vi "Initilaize Views.vi"(8 "error in (no error)":errorcluster, 11 "Example Source in":refnum<class "Example Controller Actor.lvclass">) -> (0 "error out":errorcluster, 3 "Example Source out":refnum<class "Example Controller Actor.lvclass">)   [LabVIEW 2016, in "Example Controller Actor.lvlib" / "Example Controller Actor.lvclass"]
uses:
  Example Controller Actor.lvclass
  C:/Projects/Shared Libraries/Event Actors/Controller Actor/Controller Actor.lvclass
  Example View Actor/Example View Actor/Example View Actor.lvclass
  C:/Projects/Shared Libraries/Event Actors/View Actor/View Actor.lvclass
  View Actor/View Actor.lvclass/View Actor.ctl
  View Actor/properties/Write Name.vi
  Controller Actor/Controller Actor.lvclass
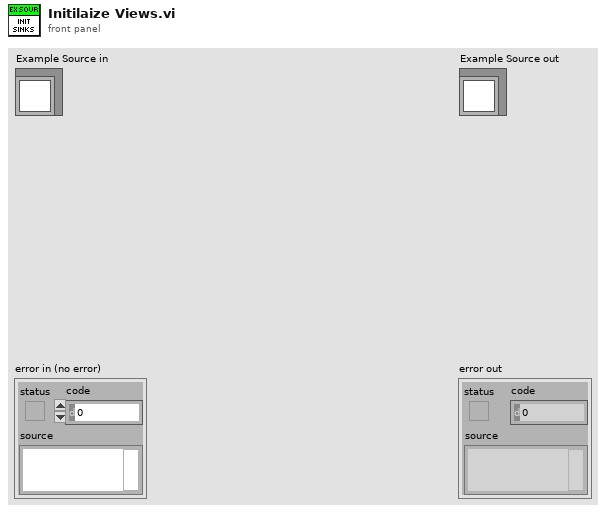
[diagram p1: front panel]
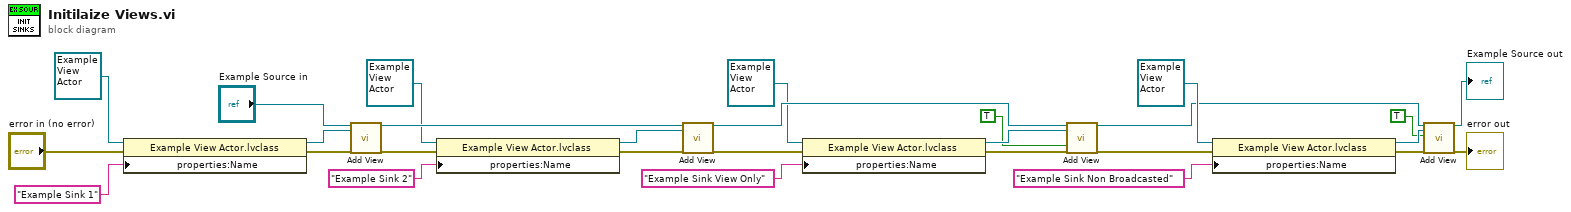
[diagram p0: block diagram]
diagram:
  n1 = property class="Example View Actor.lvclass"(reference=refnum<class "Example View Actor.lvclass"> refnum ("Alternative Example Sink.lvlib:Alternative Example Sink.lvclass"), error in="error in (no error)", "properties:Name"="Example Sink 1" ("Debug Alias")) -> (reference out=w27:refnum<class "Example View Actor.lvclass">, error out=w24:errorcluster)
  n2 = call "Add View.vi"("Controller Actor in"="Example Source in", "View Actor"=w27, "error in (no error)"=w24) -> ("Controller Actor out"=w23:refnum<class "Example Controller Actor.lvclass">, "error out"=w16:errorcluster)  [unwired: 15 in]
  n3 = property class="Example View Actor.lvclass"(reference=refnum<class "Example View Actor.lvclass"> refnum ("Alternative Example Sink.lvlib:Alternative Example Sink.lvclass"), error in=w16, "properties:Name"="Example Sink 2" ("Debug Alias")) -> (reference out=w18:refnum<class "Example View Actor.lvclass">, error out=w15:errorcluster)
  n4 = call "Add View.vi"("Controller Actor in"=w23, "View Actor"=w18, "error in (no error)"=w15) -> ("Controller Actor out"=w22:refnum<class "Example Controller Actor.lvclass">, "error out"=w14:errorcluster)  [unwired: 15 in]
  n5 = property class="Example View Actor.lvclass"(reference=refnum<class "Example View Actor.lvclass"> refnum ("Alternative Example Sink.lvlib:Alternative Example Sink.lvclass"), error in=w14, "properties:Name"="Example Sink View Only" ("Debug Alias")) -> (reference out=w17:refnum<class "Example View Actor.lvclass">, error out=w13:errorcluster)
  n6 = call "Add View.vi"("Controller Actor in"=w22, "View Actor"=w17, "Receive Only (F)"=TRUE, "error in (no error)"=w13) -> ("Controller Actor out"=w5:refnum<class "Example Controller Actor.lvclass">, "error out"=w4:errorcluster)  [unwired: 14 in]
  n7 = property class="Example View Actor.lvclass"(reference=refnum<class "Example View Actor.lvclass"> refnum ("Alternative Example Sink.lvlib:Alternative Example Sink.lvclass"), error in=w4, "properties:Name"="Example Sink Non Broadcasted" ("Debug Alias")) -> (reference out=w8:refnum<class "Example View Actor.lvclass">, error out=w7:errorcluster)
  n8 = call "Add View.vi"("Controller Actor in"=w5, "View Actor"=w8, "Exclude From Broadcast (F)"=TRUE, "error in (no error)"=w7) -> ("Controller Actor out"=→"Example Source out":refnum<class "Example Controller Actor.lvclass">, "error out"=→"error out":errorcluster)  [unwired: 14 in]
